vi "TeleopControls.vi"(0 "SteeringWheelDefRef":T1, 5 "JoystickDevRef":T1, 7 "CopilotDevRef":T1, 12 "ClimbIRVal":dbl) -> (4 "ActuateFrontClimb":dbl, 6 "ActuateBackClimb":dbl, 8 "ClimbDrive":dbl)   [LabVIEW 2018]
uses:
  <vilib>/Rock Robotics/WPI/Joystick/WPI_JoystickDevRef.ctl
  <vilib>/Rock Robotics/WPI/Joystick/WPI_JoystickDeviceEnum.ctl
  Swerve/SwerveGlobals.vi
  <vilib>/Rock Robotics/WPI/Utilities/WPI_GetSetVariantRefNum.vi
panel:
  in  "AutoClimb":bool
  # "Copilot controls:\nRight button: set arm out\nRight switch: hold down to release hatch from hatch catch\nLeft button: set arm in\nLeft switch: Cargo out?\nA button: lift low\nB button: lift mid\nC button: lift high\nRight joystick button: Start automated climb sequence\nRight joystick y axis: Up/down all climb actuators\nLeft joystick y axis: Move forward climbing\nPOV hat right: Up front climb actuator\nPOV hat left: Up back climb actuators"
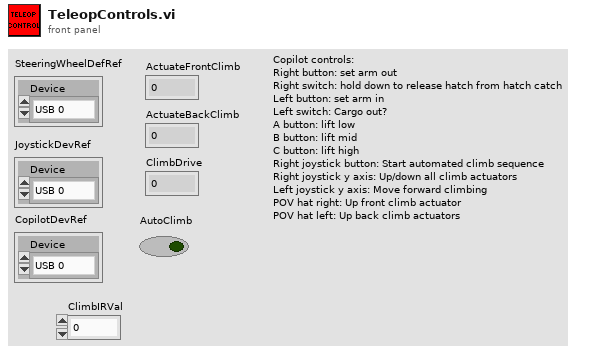
[diagram p1: front panel]
types:
  T1 = typedef "WPI_JoystickDevRef.ctl" = cluster{"Device":T2}
  T2 = typedef "WPI_JoystickDeviceEnum.ctl" = enum16{"USB 0", "USB 1", "USB 2", "USB 3", "USB 4", "USB 5"}
  T3 = typedef "WPI_CompressorDevRef.ctl" = cluster{"DevStatus":errorcluster, "Pneumatics Control Module":u8}
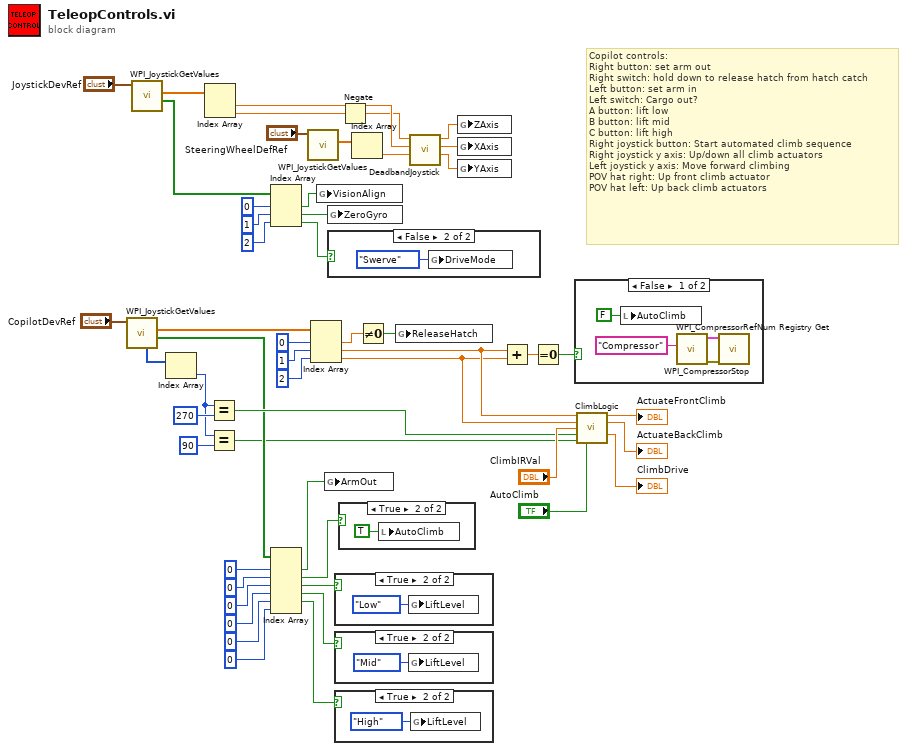
[diagram p0: block diagram]
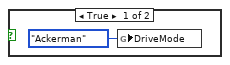
[diagram p7: hidden frame]
diagram:
  # "Copilot controls:\nRight button: set arm out\nRight switch: hold down to release hatch from hatch catch\nLeft button: set arm in\nLeft switch: Cargo out?\nA button: lift low\nB button: lift mid\nC button: lift high\nRight joystick button: Start automated climb sequence\nRight joystick y axis: Up/down all climb actuators\nLeft joystick y axis: Move forward climbing\nPOV hat right: Up front climb actuator\nPOV hat left: Up back climb actuators"
  n1 = call <vilib>:"WPI_JoystickGetValues.vi"("JoystickDevRef"="CopilotDevRef") -> ("Buttons"=w3:bool[], "Axes"=w34:dbl[], "POVs"=w8:i16[])  [unwired: 6 in, 2 out]
  n2 = call <vilib>:"WPI_JoystickGetValues.vi"("JoystickDevRef"="JoystickDevRef") -> ("Buttons"=w49:bool[], "Axes"=w51:dbl[])  [unwired: 6 in, 3 out]
  n3 = Index Array(array=w8) -> (element=w5:i16)  [unwired: 1 in]
  n4 = Index Array(array=w51) -> (element #1=w36:dbl, element #2=w50:dbl)  [unwired: 2 in]
  n5 = Equal?(x=w5, y=i16 270) -> (x = y?=w4:bool)
  n6 = Equal?(x=w5, y=i16 90) -> (x = y?=w2:bool)
  n7 = Index Array(array=w49, index #1=0 ("index"), index #2=1 ("index"), index #3=2 ("index")) -> (element #1=w42:bool, element #2=w23:bool, element #3=w43:bool)
  n8 = Index Array(array=w3, index #1=0 ("index"), index #2=0 ("index"), index #3=0 ("index"), index #4=0 ("index"), index #5=0 ("index"), index #6=0 ("index")) -> (element #1=w21:bool, element #2=w20:bool, element #3=w19:bool, element #4=w18:bool, element #5=w17:bool)  [unwired: 1 out]
  n9 = call <vilib>:"WPI_JoystickGetValues.vi"("JoystickDevRef"="SteeringWheelDefRef") -> ("Axes"=w52:dbl[])  [unwired: 6 in, 4 out]
  n10 = Index Array(array=w34, index #1=0 ("index"), index #2=1 ("index"), index #3=2 ("index")) -> (element #1=w35:dbl, element #2=w11:dbl, element #3=w10:dbl)
  n11 = global write "SwerveGlobals.vi" "VisionAlign"(w42) -> ()
  n12 = global write "SwerveGlobals.vi" "ArmOut"(w21) -> ()
  n13 = global write "SwerveGlobals.vi" "ZeroGyro"(w23) -> ()
  n14 = case shown="False" w43 {
    frame True {
      n15 = global write "SwerveGlobals.vi" "DriveMode"(enum16{"Swerve", "Ackerman"}."Ackerman" ("DriveMode")) -> ()
    }
    frame False {
      n16 = global write "SwerveGlobals.vi" "DriveMode"(enum16{"Swerve", "Ackerman"}."Swerve" ("DriveMode")) -> ()
    }
  }
  n17 = case shown="True" w19 {
    frame False {
    }
    frame True {
      n18 = global write "SwerveGlobals.vi" "LiftLevel"(enum16{"Low", "Mid", "High"}."Low" ("LiftLevel")) -> ()
    }
  }
  n19 = case shown="True" w18 {
    frame False {
    }
    frame True {
      n20 = global write "SwerveGlobals.vi" "LiftLevel"(enum16{"Low", "Mid", "High"}."Mid" ("LiftLevel")) -> ()
    }
  }
  n21 = case shown="True" w17 {
    frame False {
    }
    frame True {
      n22 = global write "SwerveGlobals.vi" "LiftLevel"(enum16{"Low", "Mid", "High"}."High" ("LiftLevel")) -> ()
    }
  }
  n23 = case shown="True" w20 {
    frame False {
    }
    frame True {
      n24 = local write "AutoClimb"(TRUE ("AutoClimb")) -> ()
    }
  }
  n25 = Negate(x=w50) -> (-x=w24:dbl)
  n26 = Index Array(array=w52) -> (element=w37:dbl)  [unwired: 1 in]
  n27 = Not Equal To 0?(x=w35) -> (x != 0?=w22:bool)
  n28 = global write "SwerveGlobals.vi" "ReleaseHatch"(w22) -> ()
  n29 = call "DeadbandJoystick.vi"("Z"=w37, "Y"=w36, "X"=w24) -> ("Z'"=w38:dbl, "Y'"=w40:dbl, "X'"=w39:dbl)  [unwired: 6 in]
  n30 = global write "SwerveGlobals.vi" "ZAxis"(w39) -> ()
  n31 = global write "SwerveGlobals.vi" "XAxis"(w40) -> ()
  n32 = global write "SwerveGlobals.vi" "YAxis"(w38) -> ()
  n33 = Add(x=w11, y=w10) -> (x+y=w1:dbl)
  n34 = Equal To 0?(x=w1) -> (x = 0?=w9:bool)
  n35 = case shown="False" w9 {
    frame False {
      n36 = local write "AutoClimb"(FALSE ("AutoClimb")) -> ()
      n37 = call <vilib>:"WPI_CompressorRefNum Registry Get.vi"("refnum name"="Compressor") -> ("error out"=w60:errorcluster, "CompressorDevRef"=w61:T3)  [unwired: 9 in]
      n38 = call <vilib>:"WPI_CompressorStop.vi"("error in (no error)"=w60, "CompressorDevRef"=w61) -> ()  [unwired: 8 in, 2 out]
    }
    frame True {
    }
  }
  n39 = call "ClimbLogic.vi"("Climb"=w11, "ClimbDriveAxis"=w10, "ClimbIRVal"="ClimbIRVal", "UpFront"=w4, "UpBack"=w2, "AutomaticClimb"="AutoClimb") -> ("ActuateFrontClimb"=→"ActuateFrontClimb":dbl, "ActuateBackClimb"=→"ActuateBackClimb":dbl, "ClimbDrive"=→"ClimbDrive":dbl)  [unwired: 7 in]
